vi "Vision 5.vi"(0 "RGB":T2, 2 "Particle Report In":T1(array[cluster]) {"Orientation" format="%.2f"; "Dimensions"."Height" format="%.2f"; "Dimensions"."Width" format="%.2f"; "Center of Mass"."Y" format="%.2f"; "Center of Mass"."X" format="%.2f"; "Bounding Rect"."Bottom" format="%.2f"; "Bounding Rect"."Right" format="%.2f"; "Bounding Rect"."Top" format="%.2f"; "Bounding Rect"."Left" format="%.2f"; "Number of Holes" format="%.2f"; "Area" format="%.2f"}, 5 "Binary":T2, 7 "FOV Angle":dbl, 9 "Target Height In Inches":dbl, 11 "Offset":dbl, 13 "Vert Theta (0.375)":dbl) -> (14 "RGB":T2, 17 "Distance":dbl, 19 "Binary":T2)   [LabVIEW 2014]
uses:
  <vilib>/vision/Image Controls.llb/IMAQ Image.ctl
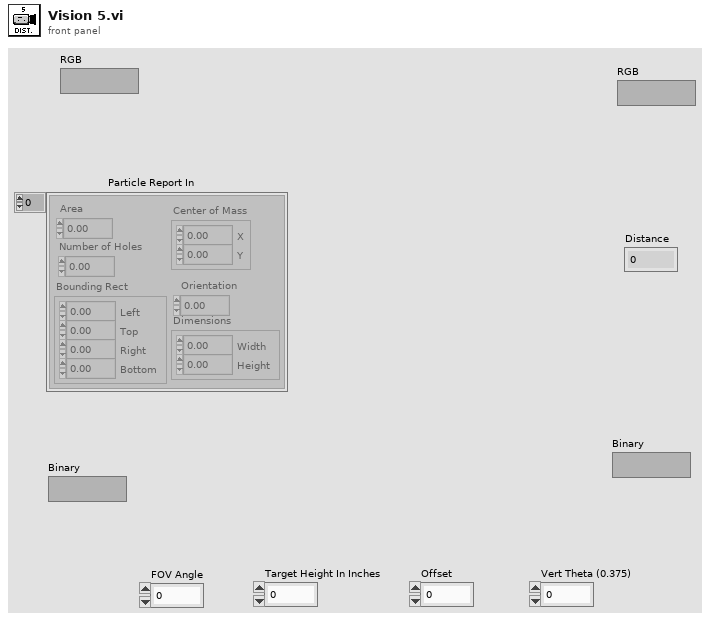
[diagram p1: front panel]
types:
  T1 = cluster{"Area":dbl, "Number of Holes":dbl, "Bounding Rect":cluster{"Left":dbl, "Top":dbl, "Right":dbl, "Bottom":dbl}, "Center of Mass":cluster{"X":dbl, "Y":dbl}, "Orientation":dbl, "Dimensions":cluster{"Width":dbl, "Height":dbl}}[]
  T2 = typedef "IMAQ Image.ctl" = refnum<image>
  T3 = cluster{"Area":dbl, "Number of Holes":dbl, "Bounding Rect":cluster{"Left":dbl, "Top":dbl, "Right":dbl, "Bottom":dbl}, "Center of Mass":cluster{"X":dbl, "Y":dbl}, "Orientation":dbl, "Dimensions":cluster{"Width":dbl, "Height":dbl}}
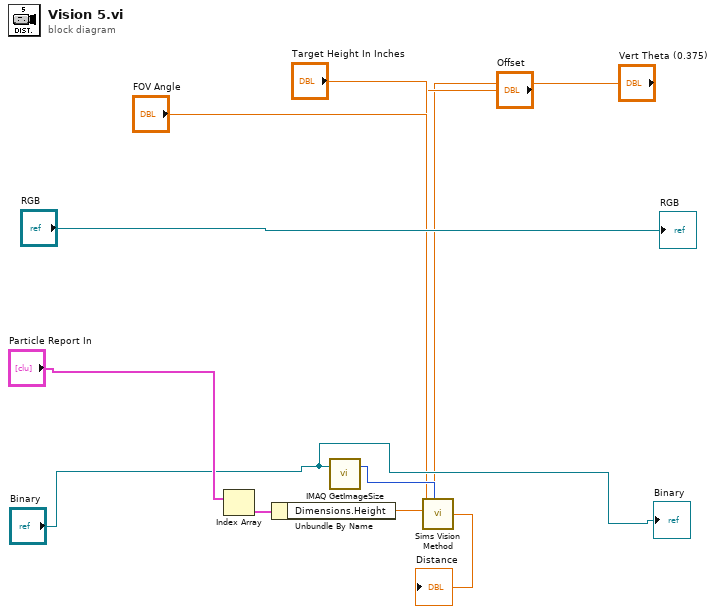
[diagram p0: block diagram]
diagram:
  n1 = Index Array(array="Particle Report In") -> (element=w11:T3)  [unwired: 1 in]
  n2 = Unbundle By Name(w11) -> ("Dimensions.Height"=w10:dbl)
  n3 = call "IMAQ GetImageSize"("Image"="Binary") -> ("Y Resolution"=w5:i32)  [unwired: 3 in, 2 out]
  n4 = call "Sims Vision Method.vi"("Vert Theta (0.375)"="Vert Theta (0.375)", "Image Hight In Pixels"=w5, "Offset"="Offset", "Target Height In Inches"="Target Height In Inches", "Target Hight In Pixels"=w10, "FOV Angle"="FOV Angle") -> ("Distance"=→"Distance":dbl)
  "Binary" <- "Binary"
  "RGB" <- "RGB"
